vi "Example Scan For Tags.vi"() -> ()   [LabVIEW 2013]
uses:
  C:/tf/play/labview/Tinkerforge.dll
panel:
  out "tag ID":u8[](array[numeric]) format="%x"
  in  "stop":bool
  out "tag type":u8
  in  "uid":string="ooK"
  in  "port":i32=4223
  in  "host":string="localhost"
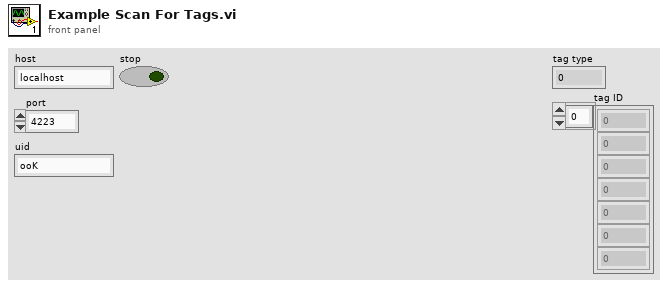
[diagram p1: front panel]
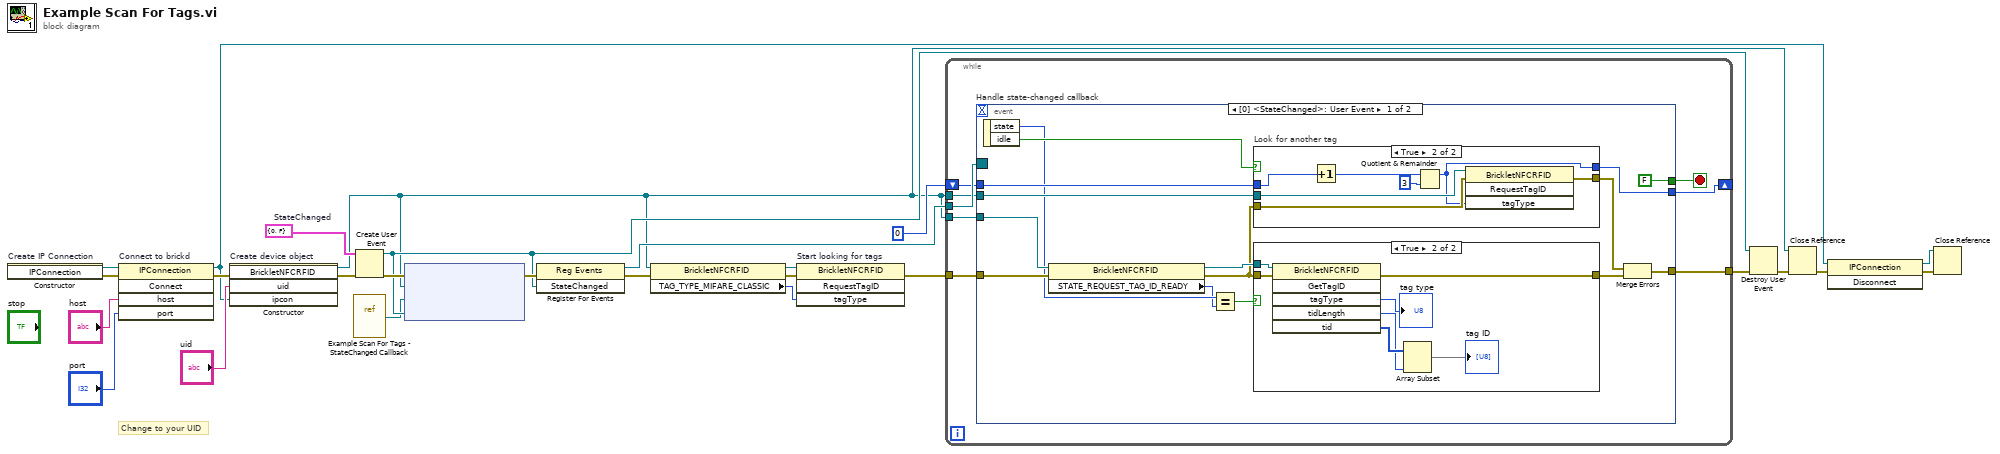
[diagram p0: block diagram]
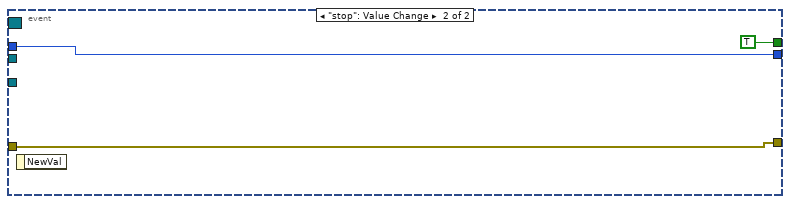
[diagram p4: hidden frame]
diagram:
  w11 = cluster{"state":u8, "idle":bool} {"state"=0, "idle"=FALSE}  # StateChanged
  # "Change to your UID"
  n1 = constructor on="Create IP Connection" class="IPConnection"() -> (reference out=w26:refnum<k24>, error out=w10:errorcluster)  [unwired: 3 in, 1 out]
  n2 = invoke on="Connect to brickd" class="IPConnection" method="Connect"(reference=w26, error in=w10, "host"="host", "port"="port") -> (reference out=w19:refnum<k24>, error out=w22:errorcluster)  [unwired: 1 in, 3 out]
  n3 = constructor on="Create device object" class="BrickletNFCRFID"(error in=w22, "uid"="uid", "ipcon"=w19) -> (reference out=w2:refnum<k24>, error out=w9:errorcluster)  [unwired: 2 in, 3 out]
  n4 = vi-ref "Example Scan For Tags - StateChanged Callback.vi"() -> ("vi reference"=w1:refnum<vi>)
  n5 = Create User Event(user event datatype=w11, error in=w9) -> (user event=w13:refnum<user-event>, error out=w17:errorcluster)
  n6 = node ("Register Event Callback")(w17, w2, w1, w13) -> (w16:errorcluster)  [unwired: 1 in, 1 out]
  n7 = register-events(error in=w16, w13) -> (reference out=w15:refnum<event-registration>, error out=w6:errorcluster)  [unwired: 1 in]
  n8 = property class="BrickletNFCRFID"(reference=w2, error in=w6) -> (reference out=w7:refnum<k24>, error out=w5:errorcluster, "TAG_TYPE_MIFARE_CLASSIC"=w4:u8)
  n9 = invoke on="Start looking for tags" class="BrickletNFCRFID" method="RequestTagID"(reference=w7, error in=w5, "tagType"=w4) -> (error out=w8:errorcluster)  [unwired: 1 in, 3 out]
  n10 = while {
    tunnel: w15 -> [w34]
    tunnel: [w33] -> w14
    tunnel: w8 -> [w32]
    shift-right: [w29] -> _
    shift-left: u8 0 -> [w30]
    tunnel: w2 -> [w28]
    tunnel: w2 -> [w27]
    stop <- w31 stop-if-true
    n11 = event "Handle state-changed callback" shown="[0] <StateChanged>: User Event" {
      selector: w34 -> [_ _]
      dyn-events: _ -> [_ _]
      timeout: _ -> [_ _]
      tunnel: [w35 w68] -> w33
      tunnel: w32 -> [w44 w68]
      tunnel: [FALSE TRUE] -> w31
      tunnel: w30 -> [w48 w67]
      tunnel: [w47 w67] -> w29
      tunnel: w28 -> [w46 _]
      tunnel: w27 -> [w43 _]
      event User Event {
        n12 = event-data() -> ("state"=w42:u8, "idle"=w45:bool)  [unwired: 1 in]
        n13 = property class="BrickletNFCRFID"(reference=w43, error in=w44) -> (reference out=w39:refnum<k24>, error out=w38:errorcluster, "STATE_REQUEST_TAG_ID_READY"=w41:u8)
        n14 = Equal?(x=w42, y=w41) -> (x = y?=w40:bool)
        n15 = case "Look for another tag" shown="True" w45 {
          tunnel: w48 -> [w59 w63]
          tunnel: [w59 w61] -> w47
          tunnel: w38 -> [w58 w66]
          tunnel: [w58 w65] -> w36
          tunnel: w46 -> [_ w64]
          frame False {
          }
          frame True {
            n16 = Increment(x=w63) -> (x+1=w62:u8)
            n17 = Quotient & Remainder(x=w62, y=u8 3) -> (x-y*floor(x/y)=w61:u8)  [unwired: 1 out]
            n18 = invoke class="BrickletNFCRFID" method="RequestTagID"(reference=w64, error in=w66, "tagType"=w61) -> (error out=w65:errorcluster)  [unwired: 1 in, 3 out]
          }
        }
        n19 = case shown="True" w40 {
          tunnel: w39 -> [_ w57]
          tunnel: w38 -> [w50 w56]
          tunnel: [w50 w55] -> w37
          frame False {
          }
          frame True {
            n20 = invoke class="BrickletNFCRFID" method="GetTagID"(reference=w57, error in=w56) -> (error out=w55:errorcluster, "tagType"=→"tag type":u8, "tidLength"=w52:u8, "tid"=w53:u8[])  [unwired: 4 in, 2 out]
            n21 = Array Subset(array=w53, length=w52) -> (→"tag ID":u8[])  [unwired: 1 in]
          }
        }
        n22 = Merge Errors(w36, w37) -> (w35:errorcluster)
      }
      event "stop": Value Change {
        n23 = event-data() -> ()  [unwired: 1 in, 1 out]
      }
    }
  }
  n24 = Destroy User Event(user event=w13, error in=w14) -> (error out=w12:errorcluster)
  n25 = Close Reference(reference=w2, error in (no error)=w12) -> (error out=w21:errorcluster)
  n26 = invoke class="IPConnection" method="Disconnect"(reference=w19, error in=w21) -> (reference out=w18:refnum<k24>, error out=w20:errorcluster)  [unwired: 1 in, 1 out]
  n27 = Close Reference(reference=w18, error in (no error)=w20) -> ()  [unwired: 1 out]
